vi "Post Initialize Action.vi"(8 "error in (no error)":errorcluster, 11 "Recipe Window in":refnum<class "Recipe Window.lvclass">) -> (0 "error out":errorcluster, 2 "Init Event Data":variant, 3 "Recipe Window out":refnum<class "Recipe Window.lvclass">)   [LabVIEW 2021, in "Recipe.lvlib" / "Recipe Window.lvclass"]
doc: "This VI is called just after the Panel Actor's UI was initialized.\n\nData wired to <b>Init Event Data</b> will be passed in the panel's \"Initialized\" user event.\n\nIf there were any initialization errors they should be handled here.\n\n----\nPlease see the following web address for additional documentation and tutorial information:\nhttp://www.mooregoodideas.com/mgi-panel-manager/\n\nAuthor: Derek Trepanier\n\nCopyright (c) 2018, Moore Good Ideas, Inc.\n\nAll rights reserved.\n\nRedistribution and use in source and binary forms, with or without modification, are permitted provided that the following conditions are met:\n\n * Redistributions of source code must retain the above copyright notice, this list of conditions and the following disclaimer.\n * Redistributions in binary form must reproduce the above copyright notice, this list of conditions and the following disclaimer in the documentation and/or other materials provided with the distribution.\n * Neither the name of Moore Good Ideas, Inc. nor the names of its contributors may be used to endorse or promote products derived from this software without specific prior written permission.\n\nTHIS SOFTWARE IS PROVIDED BY THE COPYRIGHT HOLDERS AND CONTRIBUTORS \"AS IS\" AND ANY EXPRESS OR IMPLIED WARRANTIES, INCLUDING, BUT NOT LIMITED TO, THE IMPLIED WARRANTIES OF MERCHANTABILITY AND FITNESS FOR A PARTICULAR PURPOSE ARE DISCLAIMED. IN NO EVENT SHALL THE COPYRIGHT OWNER OR CONTRIBUTORS BE LIABLE FOR ANY DIRECT, INDIRECT, INCIDENTAL, SPECIAL, EXEMPLARY, OR CONSEQUENTIAL DAMAGES (INCLUDING, BUT NOT LIMITED TO, PROCUREMENT OF SUBSTITUTE GOODS OR SERVICES; LOSS OF USE, DATA, OR PROFITS; OR BUSINESS INTERRUPTION) HOWEVER CAUSED AND ON ANY THEORY OF LIABILITY, WHETHER IN CONTRACT, STRICT LIABILITY, OR TORT (INCLUDING NEGLIGENCE OR OTHERWISE) ARISING IN ANY WAY OUT OF THE USE OF THIS SOFTWARE, EVEN IF ADVISED OF THE POSSIBILITY OF SUCH DAMAGE."
uses:
  Recipe Window.lvclass
  Recipe Window.lvclass/Recipe Window.ctl
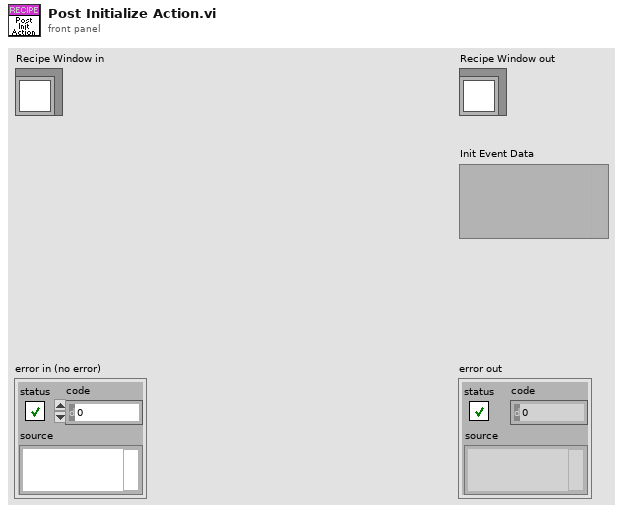
[diagram p1: front panel]
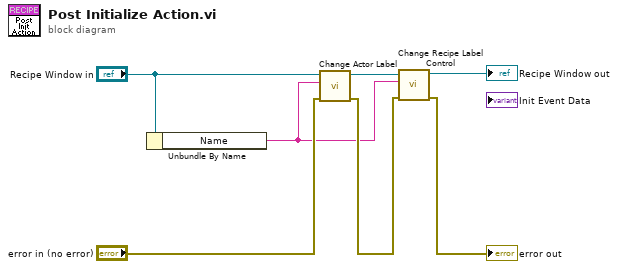
[diagram p0: block diagram]
diagram:
  n1 = Unbundle By Name("Recipe Window in") -> ("Name"=w2:string)
  n2 = call "Change Actor Label.vi"("error in (no error)"="error in (no error)", "New Label"=w2, "Recipe Window in"="Recipe Window in") -> ("error out"=w3:errorcluster, "Recipe Window out"=w1:refnum<class "Recipe Window.lvclass">)  [unwired: 7 in]
  n3 = call "Change Recipe Label Control.vi"("error in (no error)"=w3, "Label"=w2, "Recipe Window in"=w1) -> ("error out"=→"error out":errorcluster, "Recipe Window out"=→"Recipe Window out":refnum<class "Recipe Window.lvclass">)  [unwired: 7 in]
